vi "calculate_movement_ratios.vi"(11 "Robot Properties":T1) -> (3 "Robot Properties":T1)   [LabVIEW 2015]
uses:
  Robot.ctl
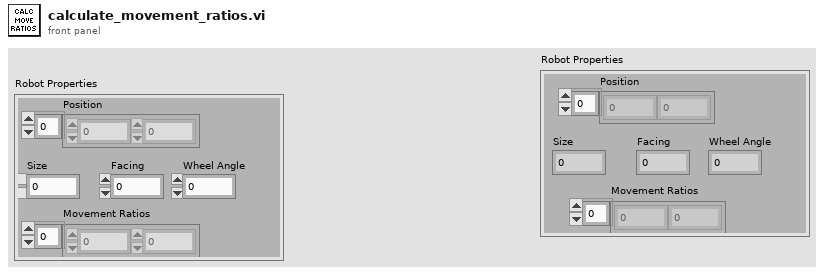
[diagram p1: front panel]
types:
  T1 = typedef "Robot.ctl" = cluster{"Position":dbl[], "Size":dbl, "Facing":dbl, "Movement Ratios":dbl[], "Wheel Angle":dbl}
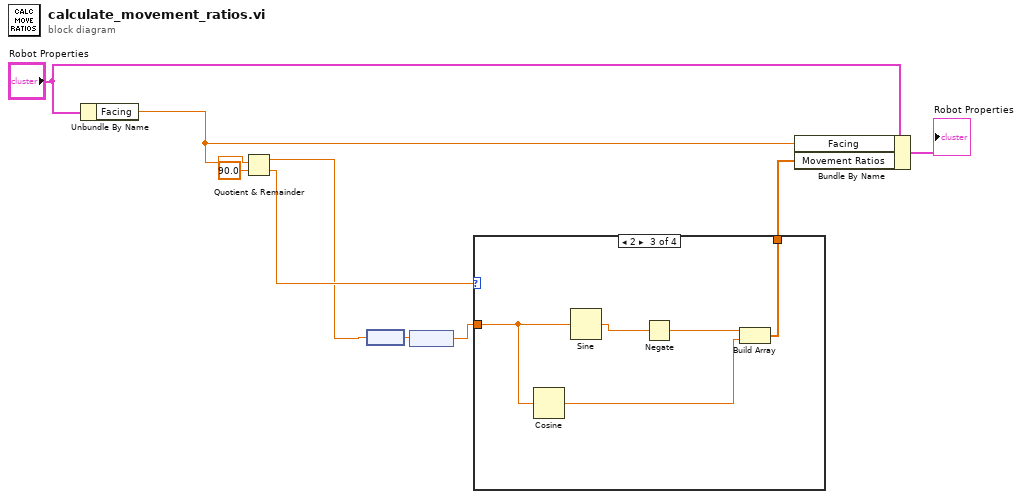
[diagram p0: block diagram]
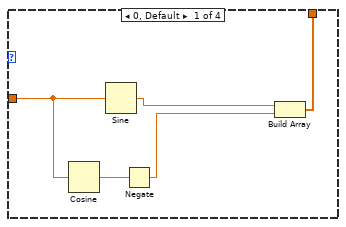
[diagram p2: hidden frame]
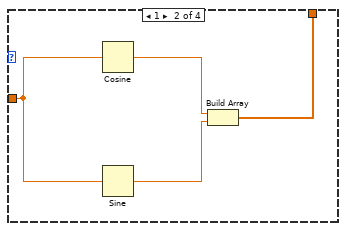
[diagram p3: hidden frame]
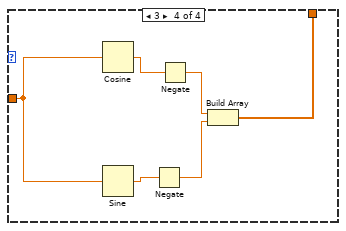
[diagram p4: hidden frame]
diagram:
  n1 = Unbundle By Name("Robot Properties") -> ("Facing"=w6:dbl)
  n2 = Quotient & Remainder(x=w6, y=90.0) -> (x-y*floor(x/y)=w2:dbl, floor(x/y)=w8:dbl)
  n3 = node(w2) -> (w1:dbl[unit])
  n4 = node(w1) -> (w3:dbl)
  n5 = case shown="2" w8 {
    tunnel: w3 -> [w14 w18 w23 w29]
    tunnel: [w13 w17 w22 w28] -> w7
    frame 0, Default {
      n6 = Cosine(x=w14) -> (cos(x)=w11:dbl)
      n7 = Sine(x=w14) -> (sin(x)=w12:dbl)
      n8 = Negate(x=w11) -> (-x=w10:dbl)
      n9 = Build Array(w12, w10) -> (w13:dbl[])
    }
    frame 1 {
      n10 = Cosine(x=w18) -> (cos(x)=w16:dbl)
      n11 = Sine(x=w18) -> (sin(x)=w15:dbl)
      n12 = Build Array(w16, w15) -> (w17:dbl[])
    }
    frame 2 {
      n13 = Cosine(x=w23) -> (cos(x)=w21:dbl)
      n14 = Sine(x=w23) -> (sin(x)=w20:dbl)
      n15 = Negate(x=w20) -> (-x=w19:dbl)
      n16 = Build Array(w19, w21) -> (w22:dbl[])
    }
    frame 3 {
      n17 = Cosine(x=w29) -> (cos(x)=w27:dbl)
      n18 = Sine(x=w29) -> (sin(x)=w25:dbl)
      n19 = Negate(x=w25) -> (-x=w24:dbl)
      n20 = Negate(x=w27) -> (-x=w26:dbl)
      n21 = Build Array(w26, w24) -> (w28:dbl[])
    }
  }
  n22 = Bundle By Name(cluster="Robot Properties", "Facing"=w6, "Movement Ratios"=w7) -> (→"Robot Properties":T1)
